vi "Pressure_Transducer_Setup.vi"(1 "Setup String":string) -> (0 "Output string":string)   [LabVIEW 2010]
uses:
  Controls/ok_button.ctl
  Controls/Pressure_Units.ctl
  Globals/Constants_global.vi
panel:
  in  "Edit Types":bool
  in  "Pressure Units":T1
  in  "10% delta P":bool caption="100% delta P"
  in  "ID number":string
  in  "Pressure Transducer type":u16(ring) items=["FCO12 Range 0-200mmH2O", "FCO12 Range 0-20mmH2O", "FCO16 Range ±200mmH2O", "FCO16 Range ±2mmH2O", "FCO332 Range 0-0.5mmH2O", "FCO332 Range 0-200mmH2O"]
  in  "OK":T2
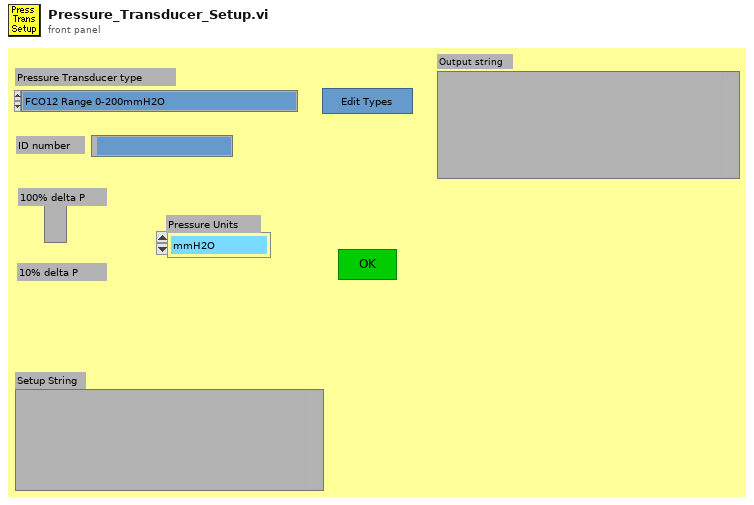
[diagram p1: front panel]
types:
  T1 = typedef "Pressure_Units.ctl" = enum16{"mmH2O", "mmHg", "Pa (N/m^2)", "mbar", "bar"}
  T2 = typedef "ok_button.ctl" = bool
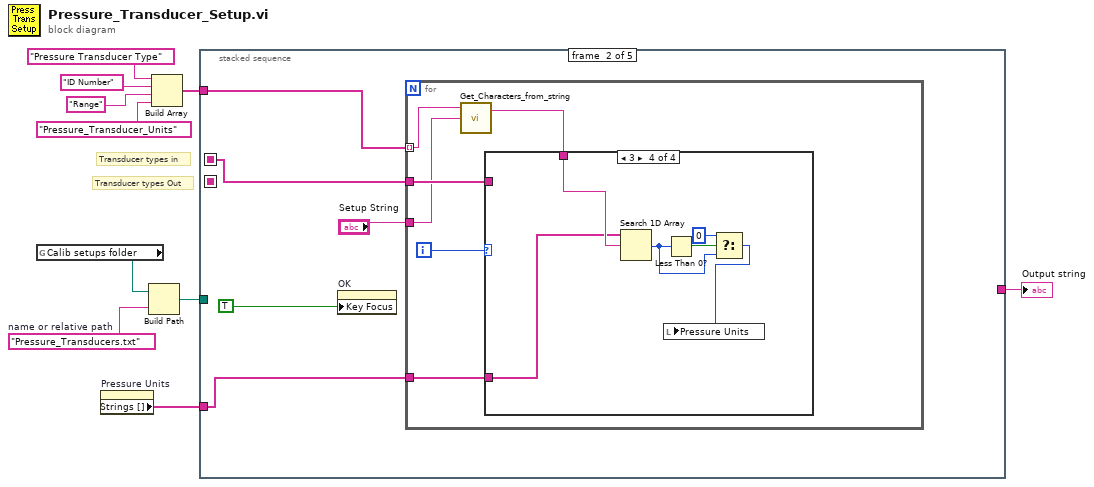
[diagram p0: block diagram]
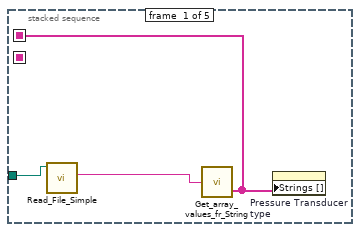
[diagram p2: hidden frame]
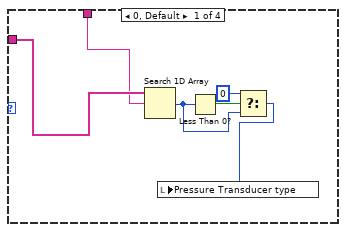
[diagram p3: hidden frame]
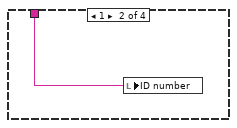
[diagram p4: hidden frame]
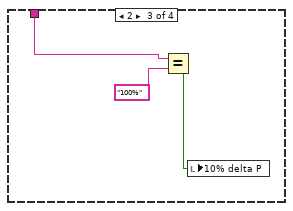
[diagram p5: hidden frame]
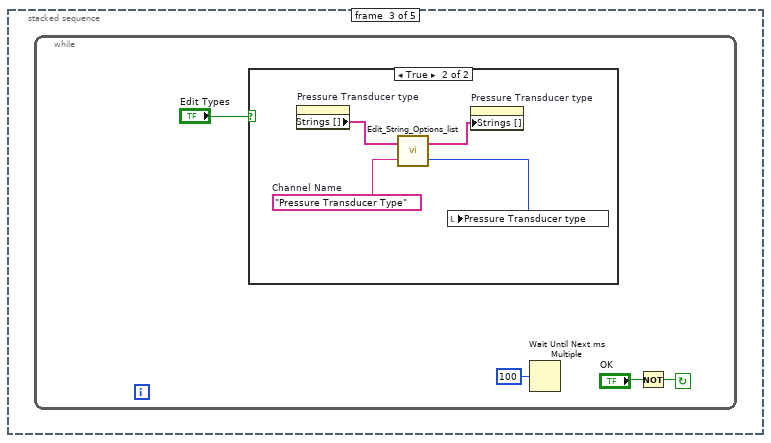
[diagram p6: hidden frame]
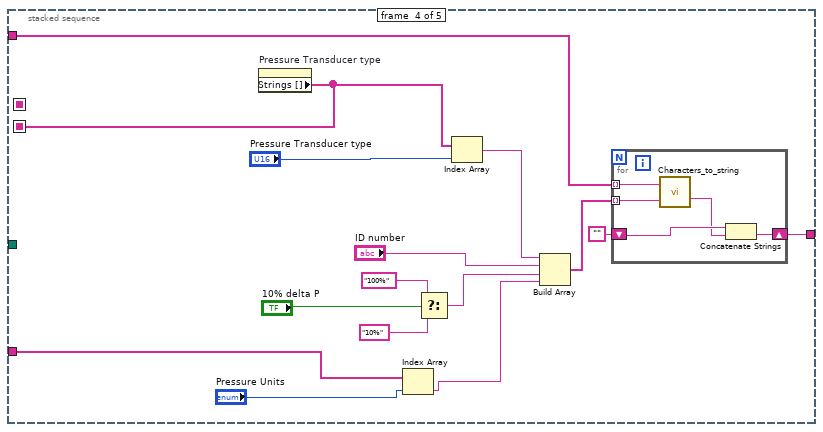
[diagram p8: hidden frame]
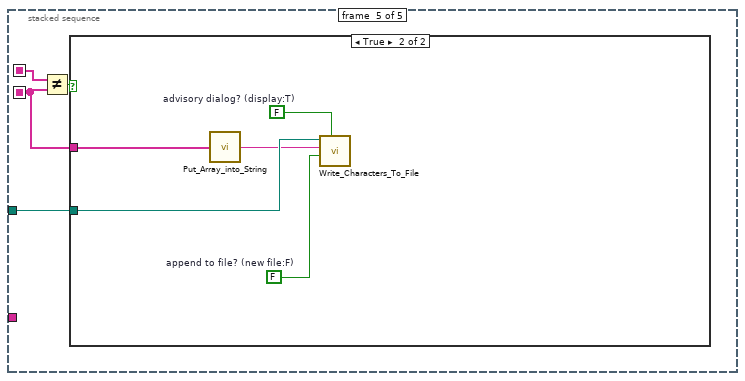
[diagram p9: hidden frame]
diagram:
  w4 = "Pressure_Transducers.txt"  # name or relative path
  # "Transducer types Out"
  # "Transducer types in"
  n1 = global read "Constants_global.vi" "Calib setups folder"() -> (w5:path)
  n2 = property on="Pressure Units" class="Enum (strict)"() -> ("Strings []"=w1:string[])  [unwired: 2 in, 2 out]
  n3 = Build Path(base path=w5, name or relative path=w4) -> (appended path=w3:path)
  n4 = Build Array("Pressure Transducer Type", "ID Number", "Range", "Pressure_Transducer_Units") -> (w7:string[])
  n5 = stacked-sequence {
    seq-local: [w11 _ _ _ _] -> [_ w15 _ _ w72]
    seq-local: [_ _ _ w50 _] -> [_ _ _ _ w70]
    tunnel: [_ _ _ w58 _] -> w10
    tunnel: w7 -> [_ w17 _ w57 _]
    tunnel: w3 -> [w13 _ _ _ w69]
    tunnel: w1 -> [_ w14 _ w49 _]
    frame #0 {
      n6 = call "Read_File_Simple.vi"("Filename"=w13) -> ("string"=w12:string)  [unwired: 2 in, 7 out]
      n7 = call "Get_array_values_fr_String.vi"("String Value"=w12) -> ("String array"=w11:string[])  [unwired: 1 out]
      n8 = property on="Pressure Transducer type" class="Ring (strict)"("Strings []"=w11) -> ()  [unwired: 2 in, 2 out]
    }
    frame #1 {
      n9 = property on="OK" class="Bool"("Key Focus"=TRUE) -> ()  [unwired: 2 in, 2 out]
      n10 = for {
        tunnel: "Setup String" -> [w21]
        tunnel: w15 -> [w23]
        tunnel: w17 -> [w22] mode=indexing
        tunnel: w14 -> [w19]
        i -> [w24]
        n11 = call "Get_Characters_from_string.vi"("Input string"=w21, "Variable name"=w22) -> ("Value"=w20:string)  [unwired: 1 in, 1 out]
        n12 = case shown="3" w24 {
          tunnel: w23 -> [w30 _ _ _]
          tunnel: w20 -> [w29 w31 w33 w40]
          tunnel: w19 -> [_ _ _ w35]
          frame 0, Default {
            n13 = Search 1D Array(1D array=w30, element=w29) -> (index of element=w27:i32)  [unwired: 1 out]
            n14 = Less Than 0?(x=w27) -> (x < 0?=w28:bool)
            n15 = Select(t=0, s=w28, f=w27) -> (s? t:f=w25:i32)
            n16 = local write "Pressure Transducer type"(w25) -> ()
          }
          frame 1 {
            n17 = local write "ID number"(w31) -> ()
          }
          frame 2 {
            n18 = Equal?(x=w33, y="100%") -> (x = y?=w32:bool)
            n19 = local write "10% delta P"(w32) -> ()
          }
          frame 3 {
            n20 = Search 1D Array(1D array=w35, element=w40) -> (index of element=w38:i32)  [unwired: 1 out]
            n21 = Less Than 0?(x=w38) -> (x < 0?=w39:bool)
            n22 = Select(t=0, s=w39, f=w38) -> (s? t:f=w36:i32)
            n23 = local write "Pressure Units"(w36) -> ()
          }
        }
      }
    }
    frame #2 {
      n24 = while {
        stop <- w43 continue-if-true
        n25 = case shown="True" "Edit Types" {
          frame False {
          }
          frame True {
            w48 = "Pressure Transducer Type"  # Channel Name
            n26 = property on="Pressure Transducer type" class="Ring (strict)"() -> ("Strings []"=w45:string[])  [unwired: 2 in, 2 out]
            n27 = call "Edit_String_Options_list.vi"("Channel Name"=w48, "String array"=w45) -> ("New Selection Index"=w46:i32, "String array Out"=w47:string[])
            n28 = local write "Pressure Transducer type"(w46) -> ()
            n29 = property on="Pressure Transducer type" class="Ring (strict)"("Strings []"=w47) -> ()  [unwired: 2 in, 2 out]
          }
        }
        n30 = Wait Until Next ms Multiple(millisecond multiple=u32 100) -> ()  [unwired: 1 out]
        n31 = Not(x="OK") -> (.not. x?=w43:T2)
      }
    }
    frame #3 {
      n32 = property on="Pressure Transducer type" class="Ring (strict)"() -> ("Strings []"=w50:string[])  [unwired: 2 in, 2 out]
      n33 = Index Array(array=w49, index="Pressure Units") -> (element=w51:string)
      n34 = Select(t="100%", s="10% delta P", f="10%") -> (s? t:f=w56:string)
      n35 = Index Array(array=w50, index="Pressure Transducer type") -> (element=w61:string)
      n36 = Build Array(w61, "ID number", w56, w51) -> (w60:string[])
      n37 = for {
        shift-right: [w64] -> w58
        shift-left: "" -> [w66]
        tunnel: w57 -> [w68] mode=indexing
        tunnel: w60 -> [w67] mode=indexing
        n38 = call "Characters_to_string.vi"("Characters to write"=w67, "Label for characters"=w68) -> ("Output string"=w65:string)
        n39 = Concatenate Strings(w66, w65) -> (w64:string)
      }
    }
    frame #4 {
      n40 = Not Equal?(x=w72, y=w70) -> (x != y?=w71:bool)
      n41 = case shown="True" w71 {
        tunnel: w70 -> [_ w77]
        tunnel: w69 -> [_ w76]
        frame False {
        }
        frame True {
          w73 = FALSE  # append to file? (new file:F)
          w74 = FALSE  # advisory dialog? (display:T)
          n42 = call "Put_Array_into_String.vi"("String array"=w77) -> ("String Value"=w75:string)
          n43 = call "Write_Characters_To_File.vi"("file path (dialog if empty)"=w76, "advisory dialog? (display:T)"=w74, "character string"=w75, "append to file? (new file:F)"=w73) -> ()  [unwired: 1 in, 4 out]
        }
      }
    }
  }
  "Output string" <- w10
